vi "Test Helper Loop Multiple Parallell Helper Loops.vi"(8 "error in (no error)":errorcluster, 11 "Helper Loop Test In":refnum<class "Helper Loop Test.lvclass">) -> (0 "error out":errorcluster, 3 "Helper Loop Test Out":refnum<class "Helper Loop Test.lvclass">)   [LabVIEW 2020, in "Helper Loop Test.lvclass"]
uses:
  Helper Loop Test.lvclass
  C:/Program Files (x86)/National Instruments/LabVIEW 2020/vi.lib/Asteme/LUnit/Test Case.lvclass
  Mock Process/Mock Process.lvclass
  C:/Users/anton/Documents/GitHub/Triarc-Framework/source/Framework/Process/Process.lvclass
  <vilib>/Asteme/LUnit/Test Case.lvclass/Test Case.ctl
  <vilib>/Asteme/LUnit/LUnit Assertion Result.lvclass/LUnit Assertion Result.ctl
  Framework/Process/Process.lvclass/Process.ctl
  Framework/Broadcast Event Helpers/Execution timer.vi
  <vilib>/Asteme/LUnit/Palette/Pass.vi
  <vilib>/Asteme/LUnit/Palette/Fail.vi
  <vilib>/Asteme/LUnit/Variant to string.vi
  <vilib>/Asteme/LUnit/Set Assertion Type.vi
  Framework/Process/Private/SubVIs/Wait for finish.vi
  Framework/Process/Protected/Messaging/Enqueue Message.vi
  Framework/Process/Private/SubVIs/Set Lifecycle State.vi
  Framework/Process/Public/Lifecycle/Get Lifecycle State.vi
  <vilib>/Asteme/LUnit/Add test result.vi
  <vilib>/Asteme/LUnit/LUnit Write Passed.vi
  <vilib>/Asteme/LUnit/LUnit Get Test Case.vi
  <vilib>/Asteme/LUnit/Assertion Result/LUnit Get Test Name.vi
  <vilib>/Asteme/LUnit/LUnit Write Message.vi
  <vilib>/Asteme/LUnit/LUnit Write Description.vi
  <vilib>/Asteme/LUnit/LUnit Write Assertion Type.vi
  <vilib>/Utility/error.llb/Clear Errors.vi
  <vilib>/Asteme/LUnit/Read Test Case Name.vi
  Framework/Broadcast Event Helpers/Dequeue Broadcast Message.vi
  <vilib>/Utility/Data Type/Get Type Information.vi
  <vilib>/Utility/LVClass/Get LV Class Name.vi
  <vilib>/Utility/error.llb/Error Cluster From Error Code.vi
  <vilib>/Asteme/LUnit/LUnit Assertion Result.lvclass
  Framework/Process/Process.lvclass
  <vilib>/Asteme/LUnit/Test Case.lvclass
  C:/Users/anton/Documents/GitHub/Triarc-Framework/source/Framework/Base/Base.lvclass
  C:/Users/anton/Documents/GitHub/Triarc-Framework/source/Framework/Configuration File/Configuration File.lvclass
  C:/Users/anton/Documents/GitHub/Triarc-Framework/source/Framework/Configuration/Configuration.lvclass
  C:/Users/anton/Documents/GitHub/Triarc-Framework/source/Framework/Error Handler Interface/Error Handler Interface.lvclass
  C:/Users/anton/Documents/GitHub/Triarc-Framework/source/Framework/Logging/Logging.lvclass
  C:/Users/anton/Documents/GitHub/Triarc-Framework/source/Framework Test/Mock Process/Mock Process.lvclass
  C:/Users/anton/Documents/GitHub/Triarc-Framework/source/Framework/Async Handler/Async Handler.lvclass
  C:/Users/anton/Documents/GitHub/Triarc-Framework/source/Framework/Helper Loop/Helper Loop.lvclass
  C:/Users/anton/Documents/GitHub/Triarc-Framework/source/Framework Test/Helper Loop Test/Helper Loop Test.lvclass
  Framework/Broadcast Event Helpers/Broadcast Event Helpers.lvlib
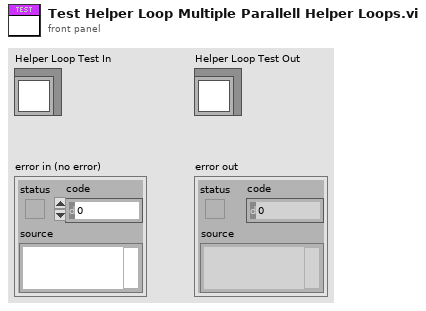
[diagram p1: front panel]
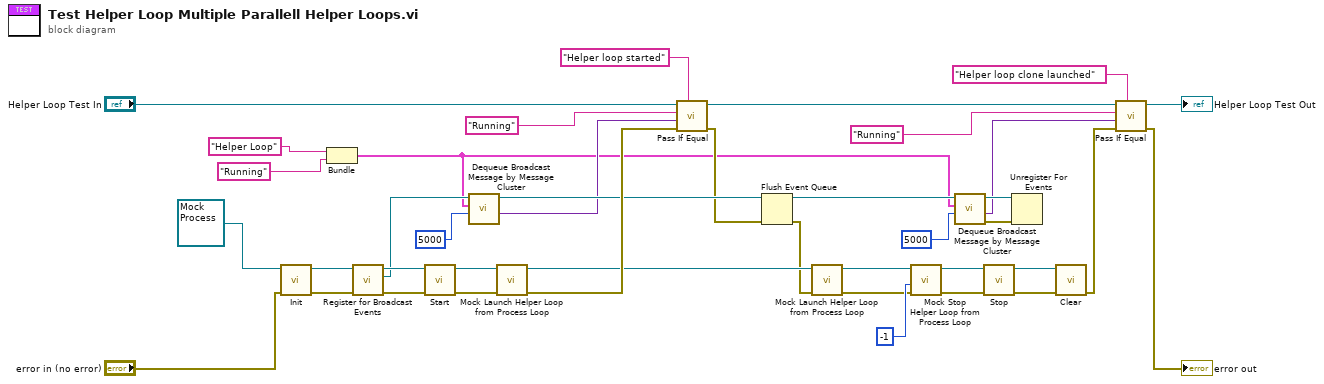
[diagram p0: block diagram]
diagram:
  n1 = call-dynamic "Init.vi"("error in (no error)"="error in (no error)", "Mock Process In"=refnum<class "Mock Process.lvclass"> refnum) -> ("error out"=w40:errorcluster, "Mock Process Out"=w20:refnum<class "Mock Process.lvclass">)  [unwired: 8 in]
  n2 = Bundle("y"="Helper Loop", "Description"="Running") -> (w1:cluster{"y":string, "Description":string})  [unwired: 1 in]
  n3 = call "Register for Broadcast Events.vi"("error in (no error)"=w40, "Process In"=w20) -> ("error out"=w21:errorcluster, "Event Registration Refnum Out"=w16:refnum<event-registration>, "Process Out"=w19:refnum<class "Mock Process.lvclass">)  [unwired: 7 in]
  n4 = call "Start.vi"("error in (no error)"=w21, "Process In"=w19) -> ("error out"=w38:errorcluster, "Process Out"=w39:refnum<class "Mock Process.lvclass">)  [unwired: 7 in, 1 out]
  n5 = call "Dequeue Broadcast Message by Message Cluster.vi"("Timeout (-1)"=5000, "Message"=w1, "Event Registration Refnum"=w16) -> ("Message Data"=w5:variant, "Event Registration Refnum Out"=w13:refnum<event-registration>)  [unwired: 4 in, 3 out]
  n6 = call "Mock Launch Helper Loop from Process Loop.vi"("error in (no error)"=w38, "Mock Process in"=w39) -> ("error out"=w27:errorcluster, "Mock Process out"=w26:refnum<class "Mock Process.lvclass">)  [unwired: 8 in]
  n7 = call <vilib>:"Pass If Equal.vi"("Description"="Helper loop started", "error in (no error)"=w27, "Actual"=w5, "Expected"="Running", "Test Case In"="Helper Loop Test In") -> ("error out"=w12:errorcluster, "Test Case Out"=w29:refnum<class "Helper Loop Test.lvclass">)  [unwired: 5 in]
  n8 = Flush Event Queue(0:w13, 3:w12) -> (8:w10:refnum<event-registration>, 11:w11:errorcluster)  [unwired: 4 in, 1 out]
  n9 = call "Mock Launch Helper Loop from Process Loop.vi"("error in (no error)"=w11, "Mock Process in"=w26) -> ("error out"=w17:errorcluster, "Mock Process out"=w18:refnum<class "Mock Process.lvclass">)  [unwired: 8 in]
  n10 = call "Mock Stop Helper Loop from Process Loop.vi"("error in (no error)"=w17, "timeout in ms (-1)"=-1, "Mock Process in"=w18) -> ("error out"=w24:errorcluster, "Mock Process out"=w25:refnum<class "Mock Process.lvclass">)  [unwired: 6 in, 1 out]
  n11 = call "Dequeue Broadcast Message by Message Cluster.vi"("Timeout (-1)"=5000, "Message"=w1, "Event Registration Refnum"=w10) -> ("error out"=w7:errorcluster, "Message Data"=w4:variant, "Event Registration Refnum Out"=w6:refnum<event-registration>)  [unwired: 4 in, 2 out]
  n12 = call "Stop.vi"("error in (no error)"=w24, "Process In"=w25) -> ("error out"=w37:errorcluster, "Process Out"=w22:refnum<class "Mock Process.lvclass">)  [unwired: 7 in, 1 out]
  n13 = Unregister For Events(event registration refnum=w6, error in=w7) -> ()  [unwired: 1 out]
  n14 = call-dynamic "Clear.vi"("error in (no error)"=w37, "Mock Process In"=w22) -> ("error out"=w36:errorcluster)  [unwired: 9 in]
  n15 = call <vilib>:"Pass If Equal.vi"("Description"="Helper loop clone launched", "error in (no error)"=w36, "Actual"=w4, "Expected"="Running", "Test Case In"=w29) -> ("error out"=→"error out":errorcluster, "Test Case Out"=→"Helper Loop Test Out":refnum<class "Helper Loop Test.lvclass">)  [unwired: 5 in]
